vi "HEWH PRAT Terminate Gallons.vi"(8 "Error In":errorcluster, 9 "GPM Target":T1 format="%.2f", 10 "Gallon Target in":T1 format="%.2f", 11 "Elapsed Time (sec)":dbl) -> (0 "Error Out":errorcluster, 2 "Time to Draw Water (Seconds)":T1 format="%.2f", 3 "Terminate":bool)   [LabVIEW 2016]
uses:
  Utility/Custom Pallet Controls/Custom Pallet DBL.ctl
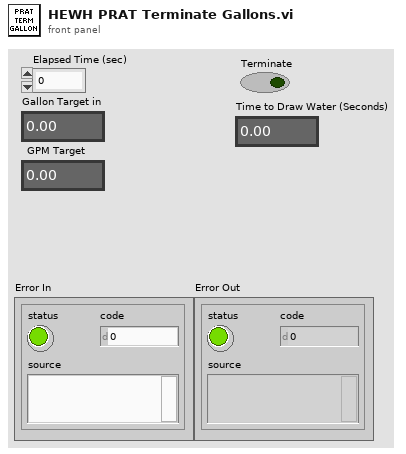
[diagram p1: front panel]
types:
  T1 = typedef "Custom Pallet DBL.ctl" = dbl
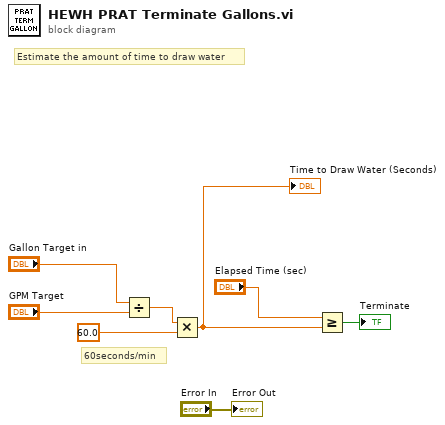
[diagram p0: block diagram]
diagram:
  # "Estimate the amount of time to draw water"
  # "60seconds/min"
  n1 = Divide(x="Gallon Target in", y="GPM Target") -> (x/y=w4:T1)
  n2 = Multiply(x=w4, y=T1 60.0) -> (x*y=w7:T1)
  "Time to Draw Water (Seconds)" <- w7
  n3 = Greater Or Equal?(x="Elapsed Time (sec)", y=w7) -> (x >= y?=→"Terminate":bool)
  "Error Out" <- "Error In"
